vi "EncoderEventExe.vi"(0 "Devices In":u64[](array[numeric]), 1 "Event Registration Refnum In":refnum<event-registration>, 5 "error in (no error)":errorcluster) -> (10 "Index":i32, 12 "Event?":bool, 13 "phid":u64, 14 "Devices Out":u64[](array[numeric]), 15 "Event Registration Refnum Out":refnum<event-registration>, 16 "Pos Change":i32, 17 "Time Change":dbl format="%.2f", 18 "Index Trigged":bool caption="Enc Index Trigged", 19 "error out":errorcluster)   [LabVIEW 2012, in "Phidget Encoder.lvlib"]
doc: "${PositionChange:Header}"
uses:
  <instrlib>/Phidgets/Phidget Encoder/Phidget Encoder.lvlib
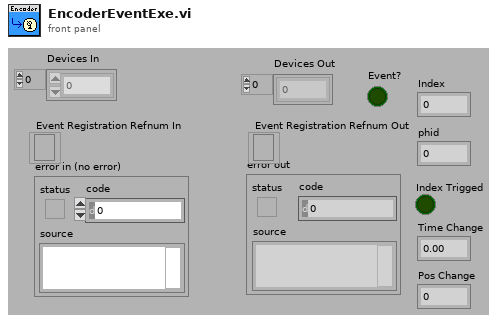
[diagram p1: front panel]
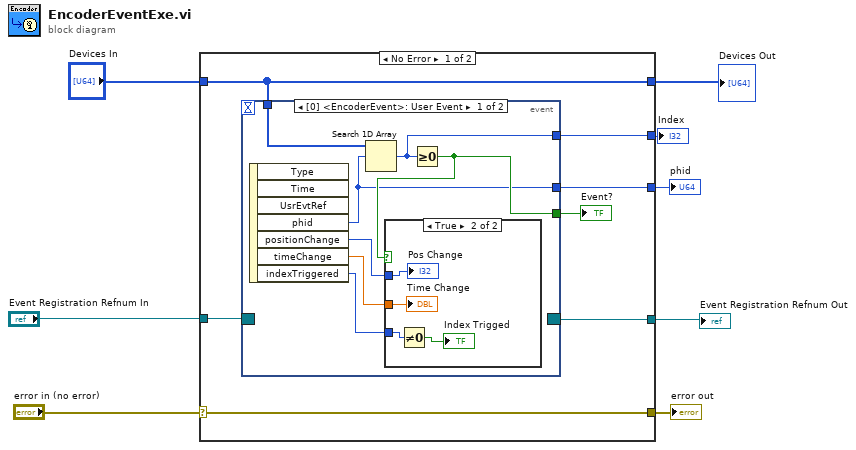
[diagram p0: block diagram]
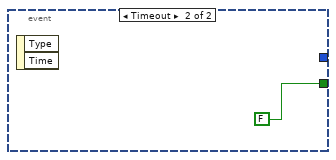
[diagram p3: hidden frame]
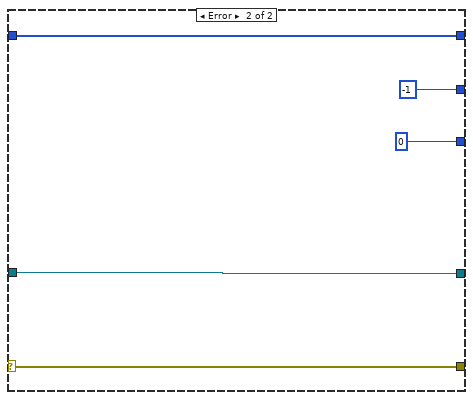
[diagram p4: hidden frame]
diagram:
  n1 = case shown="No Error" "error in (no error)" {
    selector: "error in (no error)" -> [w12 w32]
    tunnel: [w12 w32] -> w7
    tunnel: [w15 w31] -> w1
    tunnel: "Event Registration Refnum In" -> [w14 w31]
    tunnel: [w11 w30] -> w5
    tunnel: "Devices In" -> [w11 w30]
    tunnel: [w10 -1] -> w4
    tunnel: [w9 u64 0 ("number")] -> w3
    frame No Error {
      n2 = event shown="[0] <EncoderEvent>: User Event" {
        selector: w14 -> [_ _]
        dyn-events: [_ _] -> w15
        timeout: _ -> [_ _]
        tunnel: [w21 FALSE] -> w13
        tunnel: w11 -> [w22 _]
        tunnel: [w20 _] -> w10
        tunnel: [w16 _] -> w9
        event User Event {
          n3 = event-data() -> ("phid"=w16:u64, "positionChange"=w19:i32, "timeChange"=w18:dbl, "indexTriggered"=w17:i32)  [unwired: 1 in, 3 out]
          n4 = Search 1D Array(1D array=w22, element=w16) -> (index of element=w20:i32)  [unwired: 1 in]
          n5 = Greater Or Equal To 0?(x=w20) -> (x >= 0?=w21:bool)
          n6 = case shown="True" w21 {
            tunnel: w19 -> [_ w25]
            tunnel: w18 -> [_ w26]
            tunnel: w17 -> [_ w24]
            frame False {
            }
            frame True {
              n7 = Not Equal To 0?(x=w24) -> (x != 0?=→"Index Trigged":bool)
              "Time Change" <- w26
              "Pos Change" <- w25
            }
          }
        }
        event Timeout {
          n8 = event-data() -> ()  [unwired: 1 in, 2 out]
        }
      }
      "Event?" <- w13
    }
    frame Error {
    }
  }
  "error out" <- w7
  "Devices Out" <- w5
  "Index" <- w4
  "phid" <- w3
  "Event Registration Refnum Out" <- w1
